vi "page1.vi"() -> ()   [LabVIEW 2020]
panel:
  in  "Slide 3":dbl(knob) scale=0.0..10.0
  out "Slide 2":dbl(knob) scale=0.0..10.0
  out "Slide":dbl
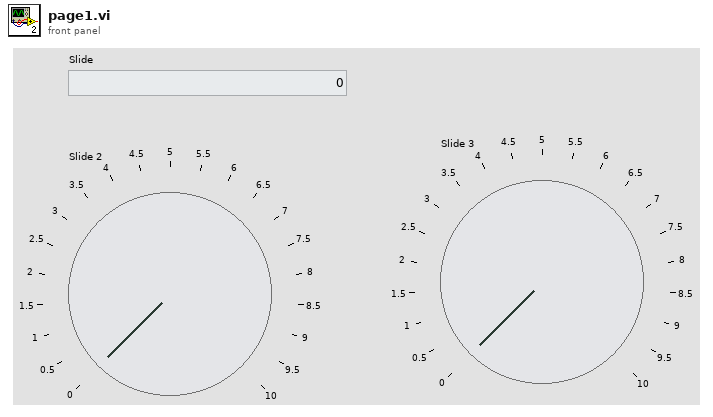
[diagram p1: front panel]
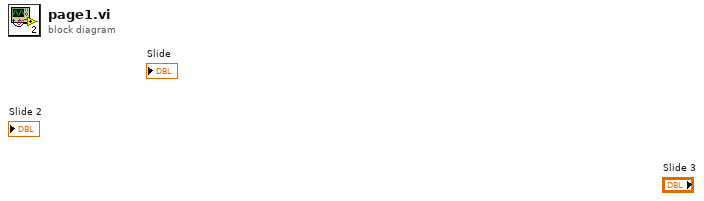
[diagram p0: block diagram]
diagram:
